vi "ValueAsBoolean.vi"(8 "error in (no error)":errorcluster, 11 "Parameter":string="  <value><boolean>0</boolean></value>\n    ") -> (0 "error out":errorcluster, 3 "value":bool)   [LabVIEW 2009]
doc: "Convert XML-RPC Boolean to LV boolean"
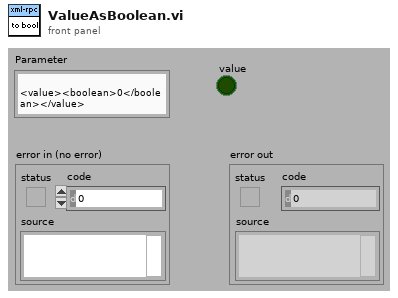
[diagram p1: front panel]
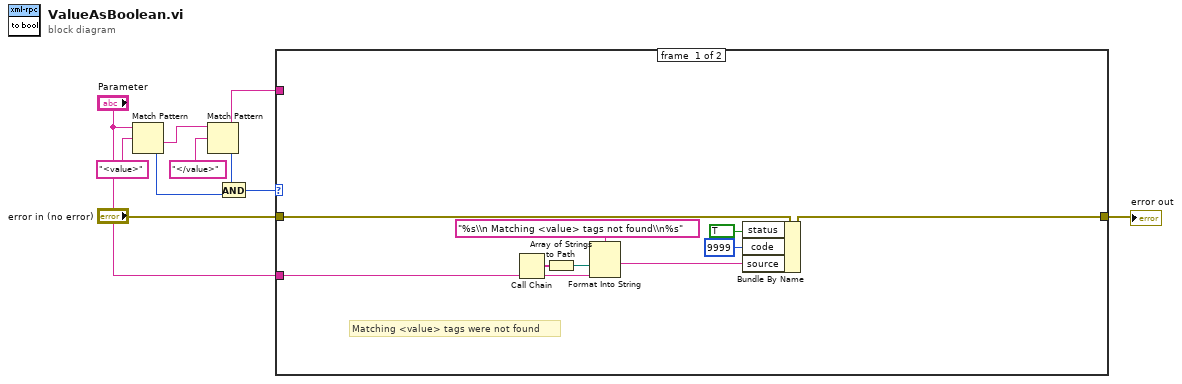
[diagram p0: block diagram]
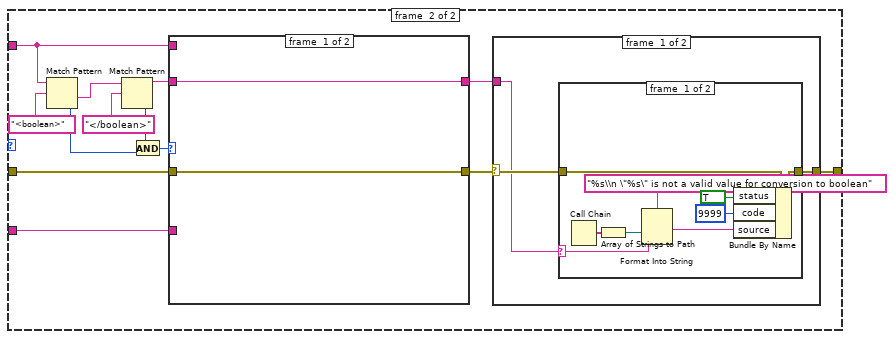
[diagram p2: hidden frame]
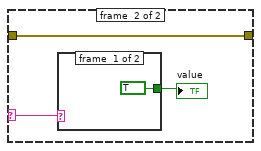
[diagram p3: hidden frame]
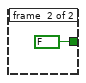
[diagram p4: hidden frame]
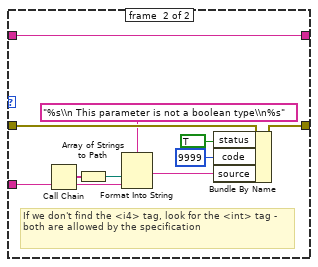
[diagram p6: hidden frame]
diagram:
  n1 = Match Pattern(string="Parameter", regular expression="<value>") -> (after substring=w9:string, offset past match=w2:i32)  [unwired: 1 in, 2 out]
  n2 = Match Pattern(string=w9, regular expression="</value>") -> (before substring=w7:string, offset past match=w3:i32)  [unwired: 1 in, 2 out]
  n3 = And(x=w3, y=w2) -> (x .and. y?=w1:i32)
  n4 = case shown="Default" w1 {
    tunnel: w7 -> [_ w29]
    tunnel: "error in (no error)" -> [w13 w27]
    tunnel: [w12 w22] -> w5
    tunnel: "Parameter" -> [w16 w26]
    frame #0 {
      # "Matching <value> tags were not found"
      n5 = Call Chain() -> (call chain=w19:string[])
      n6 = Array of Strings to Path(0:w19) -> (2:w18:path)  [unwired: 1 in]
      n7 = Format Into String(format string="%s\\n Matching <value> tags not found\\n%s", w18, w16) -> (resulting string=w11:string)  [unwired: 2 in, 1 out]
      n8 = Bundle By Name(cluster=w13, "status"=TRUE, "code"=9999, "source"=w11) -> (w12:errorcluster)
    }
    frame #1 {
      n9 = Match Pattern(string=w29, regular expression="<boolean>") -> (after substring=w31:string, offset past match=w24:i32)  [unwired: 1 in, 2 out]
      n10 = Match Pattern(string=w31, regular expression="</boolean>") -> (before substring=w28:string, offset past match=w25:i32)  [unwired: 1 in, 2 out]
      n11 = And(x=w25, y=w24) -> (x .and. y?=w23:i32)
      n12 = case shown="-1" w23 {
        tunnel: w29 -> [_ _]
        tunnel: w28 -> [w52 w53]
        tunnel: [w52 w53] -> w21
        tunnel: w27 -> [w51 w62]
        tunnel: [w51 w61] -> w20
        tunnel: w26 -> [_ w60]
        frame #0 {
        }
        frame #1 {
          # "If we don't find the <i4> tag, look for the <int> tag - both are allowed by the specification"
          n13 = Call Chain() -> (call chain=w59:string[])
          n14 = Array of Strings to Path(0:w59) -> (2:w56:path)  [unwired: 1 in]
          n15 = Format Into String(format string="%s\\n This parameter is not a boolean type\\n%s", w56, w60) -> (resulting string=w55:string)  [unwired: 2 in, 1 out]
          n16 = Bundle By Name(cluster=w62, "status"=TRUE, "code"=9999, "source"=w55) -> (w61:errorcluster)
        }
      }
      n17 = case shown="No Error" w20 {
        selector: w20 -> [w34 w50]
        tunnel: [w35 w50] -> w22
        tunnel: w21 -> [w33 _]
        frame #0 {
          n18 = case shown="Default" w33 {
            selector: w33 -> [w36 w46]
            tunnel: w34 -> [w39 w47]
            tunnel: [w38 w47] -> w35
            frame #0 {
              n19 = Call Chain() -> (call chain=w40:string[])
              n20 = Array of Strings to Path(0:w40) -> (2:w43:path)  [unwired: 1 in]
              n21 = Format Into String(format string="%s\\n \"%s\" is not a valid value for conversion to boolean", w43, w36) -> (resulting string=w44:string)  [unwired: 2 in, 1 out]
              n22 = Bundle By Name(cluster=w39, "status"=TRUE, "code"=9999, "source"=w44) -> (w38:errorcluster)
            }
            frame #1 {
              n23 = case shown="\"0\"" w46 {
                tunnel: [TRUE ("value") FALSE ("value")] -> w45
                frame #0 {
                }
                frame #1 {
                }
              }
              "value" <- w45
            }
          }
        }
        frame #1 {
          # "don't try to convert if we don't find a valid tag"
        }
      }
    }
  }
  "error out" <- w5
